vi "TemplateMethod.vi"(8 "ErrorIn":errorcluster, 9 "DummyIn":dbl, 11 "Car:Car in":refnum<class "Car.lvclass">) -> (0 "ErrorOut":errorcluster, 1 "DummyOut":dbl, 3 "Car:Car out":refnum<class "Car.lvclass">)   [LabVIEW 2021, in "Car.lvlib" / "Car.lvclass"]
uses:
  Car.lvclass
  C:/Localdata/Projects/TriekselSoft/TriekselsoftApplicationFramework/Source/.Externals/Library_YAF/YActor/YActor.lvclass
  Source/.Externals/Library_YAF/YActor/YActor.lvclass/YActor.ctl
  Source/.Externals/Library_YAF/YActor/ExeCmd_sync.vi
  319261e8-8e90-4aa5-ae36-8fd898d11326.vi
  Source/.Externals/Library_YAF/YActor/private/SendCommand.vi
  Source/.Externals/Library_YAF/YActor/private/WaitForReply.vi
  Source/.Externals/Library_YAF/YActor/private/CreateLocalVI.vi
  Source/.Externals/Library_YAF/YActor/private/ExeuteInlineVI.vi
  Source/.Externals/Library_YAF/YActor/private/GetRemoteVIRef.vi
  Source/.Externals/Library_YAF/YActor/private/GetNameOfVI.vi
  Source/.Externals/Library_YAF/YActor/QuickCast.vi
  Source/.Externals/Library_YAF/YActor/private/VINameProperty.vi
  Source/.Externals/Library_YAF/YActor/private/MessageCounter.vi
  Source/.Externals/Library_YAF/YActor/InlineReferencePool.vi
  Source/.Externals/Library_YAF/YActor/private/ExecuteVI.vi
  Source/.Externals/Library_YAF/YActor/YActor.lvclass
  Car.lvclass/Car.ctl
  C:/Localdata/Projects/TriekselSoft/TriekselsoftApplicationFramework/Source/.Externals/Library_YAF/YAFTAF/YAFTAF.lvclass
  C:/Localdata/Projects/TriekselSoft/TriekselsoftApplicationFramework/Source/.Externals/Interface_UserInterface_IFrontPanel/IFrontPanel/IFrontPanel.lvclass
  C:/Localdata/Projects/TriekselSoft/TriekselsoftApplicationFramework/Source/.Externals/Interface_TAF_IInterface/IInterface/IInterface.lvclass
  C:/Localdata/Projects/TriekselSoft/TriekselsoftApplicationFramework/Source/.Externals/Interface_Object_ICreateDestroy/ICreateDestroy/ICreateDestroy.lvclass
  C:/Localdata/Projects/TriekselSoft/TriekselsoftApplicationFramework/Source/.Externals/Interface_Object_IPersistentData/IPersistentData/IPersistentData.lvclass
  C:/Localdata/Projects/TriekselSoft/TriekselsoftApplicationFramework/Source/.Externals/Interface_TAF_ITAFObject/ITAFObject/ITAFObject.lvclass
  C:/Localdata/Projects/TriekselSoft/TriekselsoftApplicationFramework/Documentation/Project Documentation/ExampleCode/Car/Car.lvclass
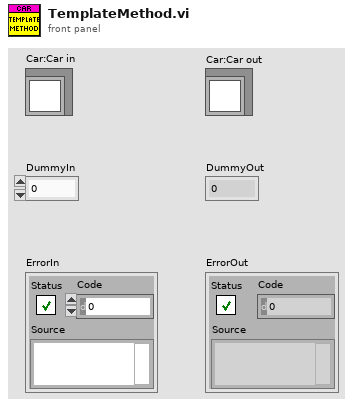
[diagram p1: front panel]
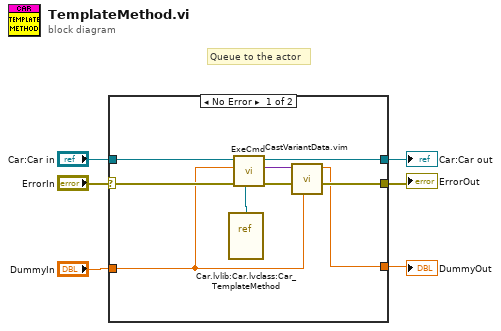
[diagram p0: block diagram]
diagram:
  # "Queue to the actor"
  n1 = case shown="No Error" "ErrorIn" {
    selector: "ErrorIn" -> [w15 w17]
    tunnel: [w13 w17] -> w5
    tunnel: [w9 w16] -> w3
    tunnel: "Car:Car in" -> [w10 w16]
    tunnel: "DummyIn" -> [w8 _]
    tunnel: [w7 _] -> w1
    frame No Error {
      n2 = vi-ref "Car.lvlib:Car.lvclass:Car_TemplateMethod.vi"() -> (w12:refnum<vi>)
      n3 = call-poly "ExeCmd.vi"("CmdVIRef"=w12, "ErrorIn"=w15, "CmdData"=w8, "YActorIn"=w10) -> ("ErrorOut"=w14:errorcluster, "ReplyData"=w11:variant, "YActorOut"=w9:refnum<class "Car.lvclass">)  [unwired: 5 in]
      n4 = call "CastVariantData.vim"("Type"=w8, "ErrorIn"=w14, "DataIn"=w11) -> ("ErrorOut"=w13:errorcluster, "DataOut"=w7:dbl)  [unwired: 7 in]
    }
    frame Error {
    }
  }
  "ErrorOut" <- w5
  "Car:Car out" <- w3
  "DummyOut" <- w1
